vi "zero channel.vi"(6 "Index":u32, 7 "Mean (Volts)":dbl format="%.5f") -> ()   [LabVIEW 2012]
uses:
  global scale array.vi
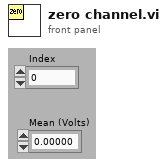
[diagram p1: front panel]
types:
  T1 = typedef "calib array.ctl" = T2[]
  T2 = typedef "conversion.ctl" = cluster{"conversion matrix":sgl[][], "units":string, "name":string, "scale type":T3, "offset (volts)":dbl, "second channel":i8, "correspondence table":T4, "offset (physical units)":dbl, "pH scale":T5, "D.O.":T6}
  T3 = typedef "scale type.ctl" = enum16{"Volts", "Polynomial", "Correspondence Table", "pH", "Dissolved Oxygen", "Quadratic"}
  T4 = typedef "correspondence table.ctl" = cluster{"physical units":dbl, "volts":dbl}[]
  T5 = typedef "pH scale.ctl" = cluster{"Buffers":cluster{"Buffer":dbl, "Calibrated":bool, "V/T":dbl}[], "Temperature":dbl}
  T6 = typedef "DO scale.ctl" = cluster{"Temperature":dbl, "K":dbl, "barometric pressure":dbl}
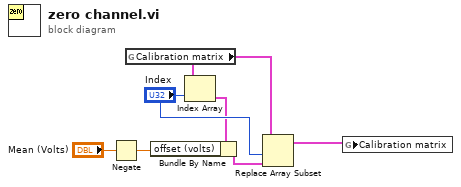
[diagram p0: block diagram]
diagram:
  n1 = Negate(x="Mean (Volts)") -> (-x=w1:dbl)
  n2 = global read "global scale array.vi" "Calibration matrix"() -> (w6:T1)
  n3 = Index Array(array=w6, index="Index") -> (element=w5:T2)
  n4 = Bundle By Name(cluster=w5, "offset (volts)"=w1) -> (w2:T2)
  n5 = Replace Array Subset(array=w6, new element=w2, index="Index") -> (w3:T1)
  n6 = global write "global scale array.vi" "Calibration matrix"(w3) -> ()
